vi "http option action.vi"(11 "application request in":T1) -> (3 "application request out":T3)   [LabVIEW 2013, in "http responder.lvclass"]
uses:
  http responder.lvclass
  http response.ctl
  http response packet type.ctl
  http request.ctl
  http method.ctl
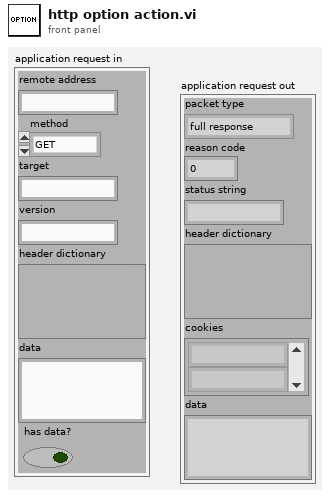
[diagram p1: front panel]
types:
  T1 = typedef "http request.ctl" = cluster{"remote address":string, "method":T2, "target":string, "version":string, "header dictionary":variant, "data":string, "has data?":bool}
  T2 = typedef "http method.ctl" = enum16{"GET", "POST", "PUT", "DELETE", "HEAD", "OPTIONS", "upgrade"}
  T3 = typedef "http response.ctl" = cluster{"packet type":T4, "reason code":u16, "status string":string, "header dictionary":variant, "cookies":string[], "data":string}
  T4 = typedef "http response packet type.ctl" = enum16{"full response", "header only", "data only", "last data"}
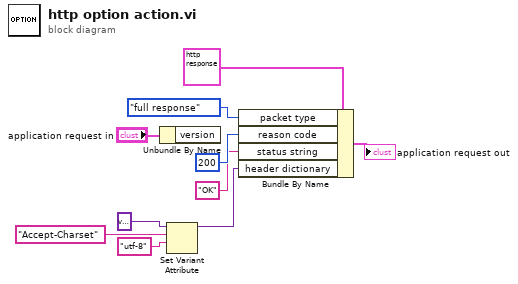
[diagram p0: block diagram]
diagram:
  n1 = Unbundle By Name("application request in") -> ()  [unwired: 1 out]
  n2 = Set Variant Attribute(Variant=variant ("variant"), name="Accept-Charset", value="utf-8" ("name")) -> (Variant out=w2:variant)  [unwired: 1 in, 2 out]
  n3 = Bundle By Name(cluster=T3 {"packet type"=enum."full response", "reason code"=0, "status string"="", "header dictionary"=variant, "cookies"=[], "data"=""} ("application request"), "packet type"=http_response_packet_type."full response", "reason code"=u16 200, "status string"="OK", "header dictionary"=w2) -> (→"application request out":T3)
